vi "Set Gain.vi"(7 "Direction":T1, 8 "error in (no error)":errorcluster, 9 "Value":sgl, 10 "Index":i32, 11 "VoiceMeeterRemote in":refnum<class "VoiceMeeterRemote.lvclass">) -> (0 "error out":errorcluster, 3 "VoiceMeeterRemote out":refnum<class "VoiceMeeterRemote.lvclass">)   [LabVIEW 2022 SP3, in "VoiceMeeterRemote.lvlib" / "VoiceMeeterRemote.lvclass"]
doc: "Sets the gain value for the specified input or output index.\n\n<b>Value</b> can be in the range of -60 to +12."
uses:
  VoiceMeeterRemote.lvclass
  Direction.ctl
  VoiceMeeterRemote.lvlib
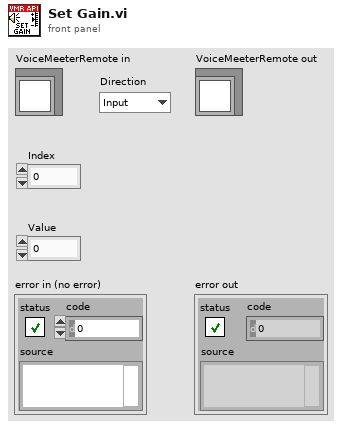
[diagram p1: front panel]
types:
  T1 = typedef "VoiceMeeterRemote.lvlib/Direction.ctl" = enum16{"Input", "Output"}
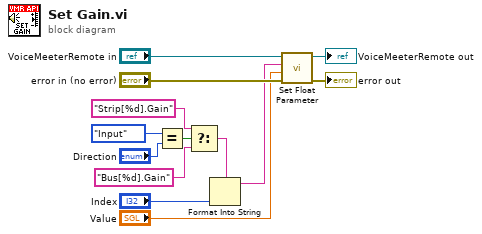
[diagram p0: block diagram]
diagram:
  n1 = Equal?(x=Direction."Input", y="Direction") -> (x = y?=w10:bool)
  n2 = Select(t="Strip[%d].Gain", s=w10, f="Bus[%d].Gain") -> (s? t:f=w4:string)
  n3 = Format Into String(format string=w4, "Index") -> (resulting string=w2:string)  [unwired: 2 in, 1 out]
  n4 = call "Set Float Parameter.vi"("error in (no error)"="error in (no error)", "Value"="Value", "Parameter Name"=w2, "VoiceMeeterRemote in"="VoiceMeeterRemote in") -> ("error out"=→"error out":errorcluster, "VoiceMeeterRemote out"=→"VoiceMeeterRemote out":refnum<class "VoiceMeeterRemote.lvclass">)  [unwired: 6 in]
